vi "ReadModuleConfiguration (SubVI).vi"(0 "Module configuration file path":path, 5 "Fiducial Mark":string(combo)="MarkB", 11 "error in (no error)":errorcluster) -> (3 "Strip pitch [um]":dbl, 4 "Width [mm]":dbl, 6 "Height [mm]":dbl, 8 "Lx":dbl, 10 "Ly":dbl, 14 "Template filename":string, 15 "error out":errorcluster)   [LabVIEW 2016]
uses:
  <vilib>/Utility/config.llb/Read Key (Double).vi
  <vilib>/Utility/config.llb/Read Key (String).vi
  <vilib>/Utility/config.llb/NI_LVConfig.lvlib
panel:
  out "Fiducial":string
  # "Fiducial distances"
  # "Module Properties"
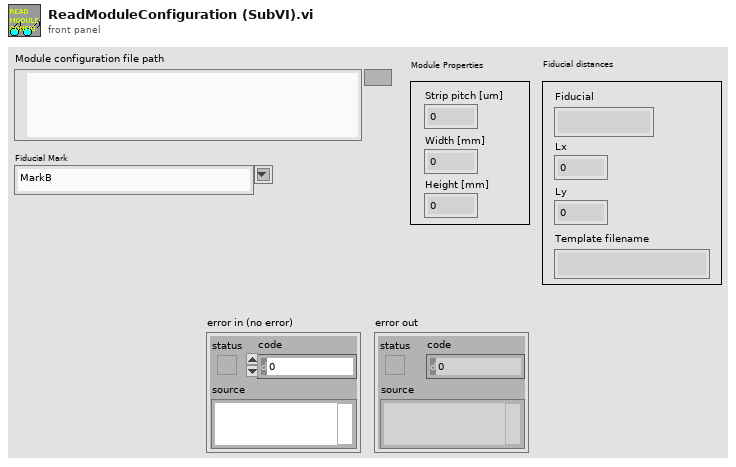
[diagram p1: front panel]
types:
  T1 = typedef "NI_LVConfig.lvlib/Config Data RefNum.ctl" = refnum<k1>
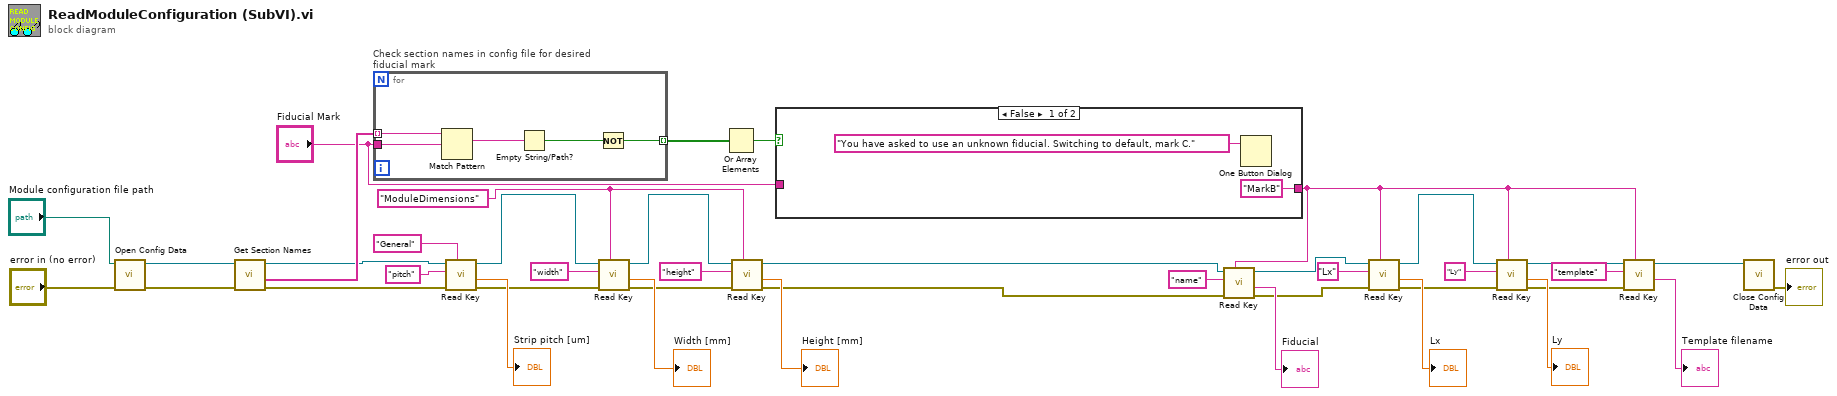
[diagram p0: block diagram]
diagram:
  w36 = "ModuleDimensions" ("section")
  n1 = call <vilib>:"Open Config Data.vi"("error in (no error)"="error in (no error)", "configuration file path"="Module configuration file path") -> ("error out"=w29:errorcluster, "refnum"=w40:T1)  [unwired: 7 in, 1 out]
  n2 = call <vilib>:"Get Section Names.vi"("error in (no error)"=w29, "refnum"=w40) -> ("error out"=w14:errorcluster, "section names"=w30:string[], "refnum out"=w23:T1)  [unwired: 7 in]
  n3 = for "Check section names in config file for desired fiducial mark" {
    tunnel: w30 -> [w45] mode=indexing
    tunnel: "Fiducial Mark" -> [w43]
    tunnel: [w42] -> w28 mode=indexing
    n4 = Match Pattern(string=w45, regular expression=w43) -> (match substring=w46:string)  [unwired: 1 in, 3 out]
    n5 = Empty String/Path?(string/path=w46) -> (empty?=w44:bool)
    n6 = Not(x=w44) -> (.not. x?=w42:bool)
  }
  n7 = call-poly <vilib>:"Read Key.vi"("section"="General", "error in (no error)"=w14, "key"="pitch", "refnum"=w23) -> ("error out"=w15:errorcluster, "value"=→"Strip pitch [um]":dbl, "refnum out"=w20:T1)  [unwired: 4 in, 1 out]
  n8 = call-poly <vilib>:"Read Key.vi"("section"=w36, "error in (no error)"=w15, "key"="width", "refnum"=w20) -> ("error out"=w16:errorcluster, "value"=→"Width [mm]":dbl, "refnum out"=w19:T1)  [unwired: 4 in, 1 out]
  n9 = Or Array Elements(Boolean array=w28) -> (logical OR=w27:bool)
  n10 = call-poly <vilib>:"Read Key.vi"("section"=w36, "error in (no error)"=w16, "key"="height", "refnum"=w19) -> ("error out"=w8:errorcluster, "value"=→"Height [mm]":dbl, "refnum out"=w9:T1)  [unwired: 4 in, 1 out]
  n11 = case shown="False" w27 {
    tunnel: "Fiducial Mark" -> [_ w49]
    tunnel: ["MarkB" ("Fiducial Mark") w49] -> w3
    frame False {
      n12 = One Button Dialog(message="You have asked to use an unknown fiducial. Switching to default, mark C.") -> ()  [unwired: 1 in, 1 out]
    }
    frame True {
    }
  }
  n13 = call-poly <vilib>:"Read Key.vi"("section"=w3, "error in (no error)"=w8, "key"="name", "refnum"=w9) -> ("error out"=w10:errorcluster, "value"=→"Fiducial":string, "refnum out"=w12:T1)  [unwired: 4 in, 1 out]
  n14 = call-poly <vilib>:"Read Key.vi"("section"=w3, "error in (no error)"=w10, "key"="Lx", "refnum"=w12) -> ("error out"=w17:errorcluster, "value"=→"Lx":dbl, "refnum out"=w25:T1)  [unwired: 4 in, 1 out]
  n15 = call-poly <vilib>:"Read Key.vi"("section"=w3, "error in (no error)"=w17, "key"="Ly", "refnum"=w25) -> ("error out"=w5:errorcluster, "value"=→"Ly":dbl, "refnum out"=w6:T1)  [unwired: 4 in, 1 out]
  n16 = call-poly <vilib>:"Read Key.vi"("section"=w3, "error in (no error)"=w5, "key"="template", "refnum"=w6) -> ("value"=→"Template filename":string, "refnum out"=w2:T1)  [unwired: 4 in, 2 out]
  n17 = call <vilib>:"Close Config Data.vi"("refnum"=w2) -> ("error out"=→"error out":errorcluster)  [unwired: 9 in, 1 out]
